vi "if_v0_v6.vi"() -> ()   [LabVIEW 2009]
panel:
  out "String":string="Solutii reale"
  out "X2":dbl=-0.27525512860841106
  out "X1":dbl=2.724744871391589
  in  "a":dbl=4.0
  in  "c":dbl=3.0
  in  "b":dbl=12.0
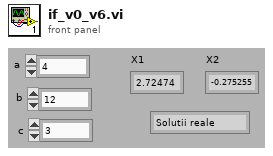
[diagram p1: front panel]
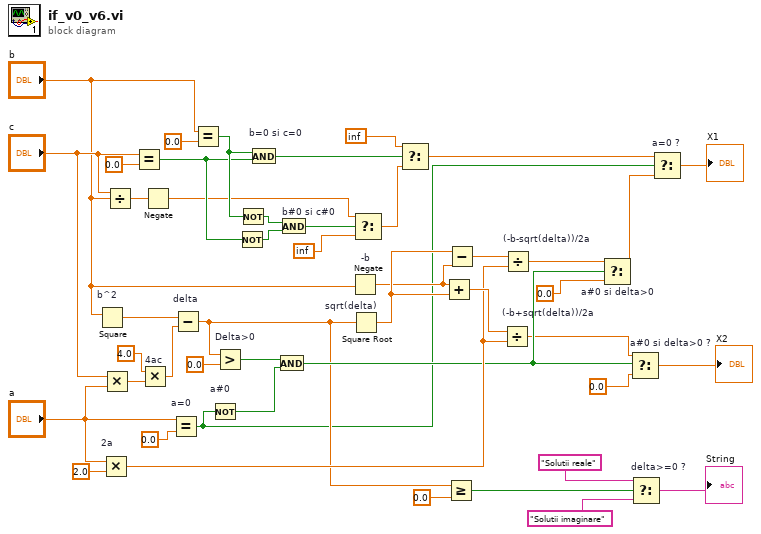
[diagram p0: block diagram]
diagram:
  n1 = Square "b^2"(x="b") -> (x^2=w28:dbl)
  n2 = Multiply "2a"(x="a", y=2.0) -> (x*y=w17:dbl)
  n3 = Multiply(x="c", y="a") -> (x*y=w30:dbl)
  n4 = Divide(x="c", y="b") -> (x/y=w36:dbl)
  n5 = Equal?(x="c", y=0.0) -> (x = y?=w39:bool)
  n6 = Multiply "4ac"(x=4.0, y=w30) -> (x*y=w27:dbl)
  n7 = Negate(x=w36) -> (-x=w35:dbl)
  n8 = Equal? "a=0"(x="a", y=0.0) -> (x = y?=w1:bool)
  n9 = Subtract "delta"(x=w28, y=w27) -> (x-y=w2:dbl)
  n10 = Equal?(x="b", y=0.0) -> (x = y?=w41:bool)
  n11 = Not "a#0"(x=w1) -> (.not. x?=w24:bool)
  n12 = Greater? "Delta>0"(x=w2, y=0.0) -> (0:w25:bool)
  n13 = Not(x=w39) -> (.not. x?=w38:bool)
  n14 = Not(x=w41) -> (.not. x?=w40:bool)
  n15 = And "b=0 si c=0"(x=w41, y=w39) -> (x .and. y?=w44:bool)
  n16 = And(x=w25, y=w24) -> (x .and. y?=w15:bool)
  n17 = And "b#0 si c#0"(x=w40, y=w38) -> (x .and. y?=w37:bool)
  n18 = Negate "-b"(x="b") -> (-x=w18:dbl)
  n19 = Square Root "sqrt(delta)"(x=w2) -> (sqrt(x)=w19:dbl)
  n20 = Select(t=w35, s=w37, f=inf) -> (s? t:f=w33:dbl)
  n21 = Select(t=inf, s=w44, f=w33) -> (s? t:f=w42:dbl)
  n22 = Add(x=w18, y=w19) -> (x+y=w20:dbl)
  n23 = Greater Or Equal?(x=w2, y=0.0) -> (x >= y?=w6:bool)
  n24 = Subtract ("-b-sqrt(delta)")(x=w19, y=w18) -> (x-y=w16:dbl)
  n25 = Divide "(-b+sqrt(delta))/2a"(x=w20, y=w17) -> (x/y=w13:dbl)
  n26 = Divide "(-b-sqrt(delta))/2a"(x=w16, y=w17) -> (x/y=w14:dbl)
  n27 = Select "a#0 si delta>0"(t=w14, s=w15, f=0.0 ("y")) -> (s? t:f=w8:dbl)
  n28 = Select "a#0 si delta>0 ?"(t=w13, s=w15, f=0.0 ("y")) -> (s? t:f=→"X2":dbl)
  n29 = Select "delta>=0 ?"(t="Solutii reale", s=w6, f="Solutii imaginare") -> (s? t:f=→"String":string)
  n30 = Select "a=0 ?"(t=w42, s=w1, f=w8) -> (s? t:f=→"X1":dbl)
